vi "Parse Data.vi"(3 "Head Channel":i16, 4 "Raw Data":dbl[](array[numeric]), 5 "Pulsar Handle":i16) -> (1 "Selected data":dbl[][](array[numeric]))   [LabVIEW 2009]
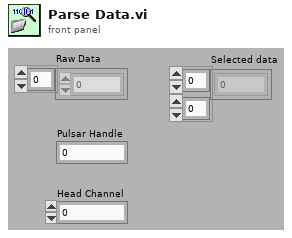
[diagram p1: front panel]
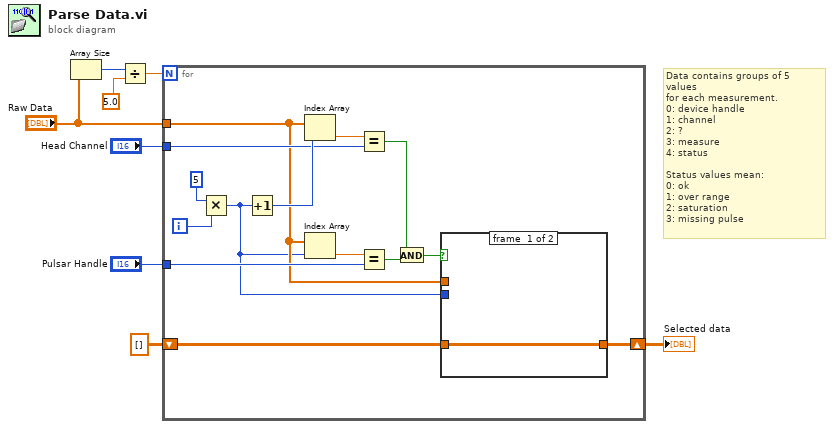
[diagram p0: block diagram]
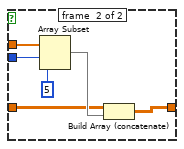
[diagram p2: hidden frame]
diagram:
  # "Data contains groups of 5 values\nfor each measurement.\n0: device handle\n1: channel\n2: ?\n3: measure\n4: status\n\nStatus values mean:\n0: ok\n1: over range\n2: saturation\n3: missing pulse"
  n1 = Array Size(array="Raw Data") -> (size(s)=w7:i32)
  n2 = Divide(x=w7, y=5.0) -> (x/y=w6:dbl)
  n3 = for {
    N: w6 -> [_]
    tunnel: "Raw Data" -> [w13]
    shift-right: [w9] -> w1
    shift-left: dbl[][] [] -> [w10]
    tunnel: "Head Channel" -> [w17]
    tunnel: "Pulsar Handle" -> [w16]
    i -> [w20]
    n4 = Multiply(x=5, y=w20) -> (x*y=w11:i32)
    n5 = Increment(x=w11) -> (x+1=w21:i32)
    n6 = Index Array(array=w13, index=w21) -> (element=w18:dbl)
    n7 = Index Array(array=w13, index=w11) -> (element=w19:dbl)
    n8 = Equal?(x=w18, y=w17) -> (x = y?=w15:bool)
    n9 = Equal?(x=w19, y=w16) -> (x = y?=w14:bool)
    n10 = And(x=w15, y=w14) -> (x .and. y?=w12:bool)
    n11 = case shown="True" w12 {
      tunnel: w13 -> [_ w29]
      tunnel: w11 -> [_ w27]
      tunnel: w10 -> [w23 w25]
      tunnel: [w23 w24] -> w9
      frame #0 {
      }
      frame #1 {
        n12 = Array Subset(array=w29, index=w27, length=5) -> (w26:dbl[])
        n13 = Build Array (concatenate)(w25, w26) -> (w24:dbl[][])
      }
    }
  }
  "Selected data" <- w1
